vi "Err_Handling.vi"() -> ()   [LabVIEW 2012, in "TB1kW_ErrorProg.lvlib"]
uses:
  TB1kW_ErrorProg.lvlib
  Control and Global/Global_Variables.vi
  Control and Global/Format_Error.ctl
  <vilib>/Utility/error.llb/DialogType.ctl
  <vilib>/Utility/miscctls.llb/LVPointTypeDef.ctl
panel:
  out "Air 100W":bool
  out "O2 100W":bool
  out "H2 CO 100W":bool
  out "N2 100W":bool
  out "H2 100W":bool
  out "MeasErr Array 100W":T1[](array[typedef])
  out "New MesErr file to load 1kW":bool
  out "Last Error/Warning":string
  in  "Show Internal Errors":bool
  out "Watch Dog":bool
  in  "Clear Hist":bool
  out "USV: No 230V":bool
  out "Air":bool
  out "O2":bool
  out "N2":bool
  out "H2":bool
  out "H2 CO":bool
  out "H2 Detected":bool
  out "Em Stop Relay":bool
  out "Em Stop":bool
  out "Error Warning History":string[][](table)
  in  "More/Less":bool
  out "MeasErr Array":T1[](array[typedef])
  in  "Em Stop":bool
  # "Pressure out of range"
  # "Dieser Cluster wird verwendet um das Measurement Error File richtig zu formatieren.\nName: Name des Eingangs, Grösse oder Wertes\nOptions: \n 00: Status des Werts: ok (0), Warnung (-1), Fehler (1)\n 01: Maximaler Wert\n 02: Maximale Dauer in der dieser Wert überschritten werden darf. [s]\n 03: spezifische optionen\nLast Chek at: Zeitpunkt an dem der Wert das letzte Mal geprüft wurde ohne dass ein Limit überschritten wured . Der Zeitpunkt wird nicht mer aktualisiert, falls ein Fehler auftritt so kann die Dauer ermittelt werden."
  # "Dieser Cluster wird verwendet um das Measurement Error File richtig zu formatieren.\nName: Name des Eingangs, Grösse oder Wertes\nOptions: \n 00: Status des Werts: ok (0), Warnung (-1), Fehler (1)\n 01: Maximaler Wert\n 02: Maximale Dauer in der dieser Wert überschritten werden darf. [s]\n 03: spezifische optionen\nLast Chek at: Zeitpunkt an dem der Wert das letzte Mal geprüft wurde ohne dass ein Limit überschritten wured . Der Zeitpunkt wird nicht mer aktualisiert, falls ein Fehler auftritt so kann die Dauer ermittelt werden."
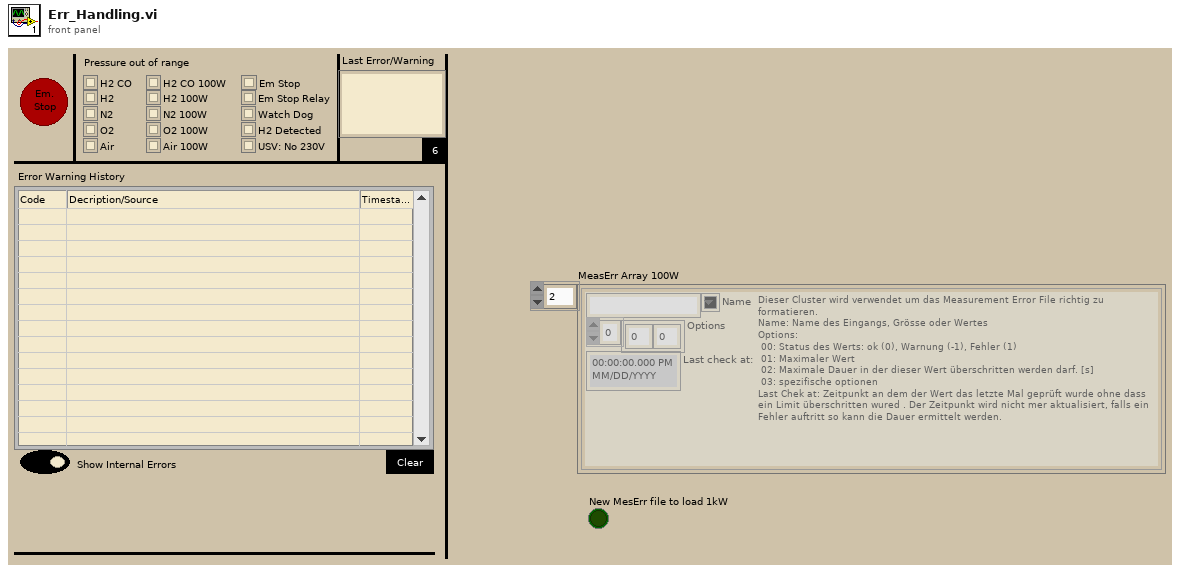
[diagram p1: front panel]
types:
  T1 = typedef "TB1kW_Controls.lvlib/Format_Error.ctl" = cluster{"Name":string, "Options":dbl[], "Last check at:":timestamp}
  T2 = typedef "LVPointTypeDef.ctl" = cluster{"Horizontal":i16, "Vertical":i16}
  T3 = cluster{"Em. Button pressed":bool, "Em. Relay In":bool, "H2 detected":bool, "Watch Dog In":bool, "P_H2 not OK (1)":bool, "P_H2 not OK (2)":bool, "P_N2 not OK (1)":bool, "P_N2 not OK (2)":bool, "P_H2CO not OK (1)":bool, "P_H2CO not OK (2)":bool, "P_O2 not OK (1)":bool, "P_O2 not OK (2)":bool, "P_Air not OK (1)":bool, "P_Air not OK (2)":bool, "I/O 14 MUX":bool, "I/O 15 MUX":bool, "I/O 5":bool, "EM Stop Relay Out":bool, "Watch Dog Out":bool, "USV: No ~230V":bool}
  T4 = cluster{"f1":bool, "f2":bool, "f2":bool, "f3":bool, "New MesErr file to load":bool, "New Command file to load":bool, "f6":bool, "f7":bool, "New MesErr file to load 100W":bool, "New Command file to load 100W":bool}
  T5 = cluster{"Internal Error 1kW":bool, "Test Error 1kW":bool, "Shut down test":bool, "Terminate programm":bool, "Set secure state":bool, "Test is running":bool, "Flush after Error 1kW":bool, "f07":bool, "f08":bool, "Command file created":bool, "f10":bool, "f11":bool, "f12":bool, "f13":bool, "Logging":bool, "Is Measuring Cell Imp.":bool, "Test is running 100W":bool, "Command file created 100W":bool, "Shut down test 100W":bool, "Logging 100W":bool, "Internal Error 100W":bool, "Test Error 100W":bool, "Internal Error":bool, "Set secure state 100W":bool, "Flush after Error 100W":bool, "Init_Dnet":bool, "Use Stopsequenz 1kW":bool, "Use Stopsequenz 100W":bool, "Do Stopsequenz 1kW":bool, "Do Stopsequenz 100W":bool}
  T6 = typedef "Semaphore RefNum" = refnum<k1>
  T7 = typedef "DialogType.ctl" = u16
  T8 = typedef "TB1kW_Controls.lvlib/Test_Properties.ctl" = cluster{"Cell Properties":T9, "Time":T10, "Flow N2 to Ox [Nl/min]":dbl, "Flow N2 to Fuel [Nl/min]":dbl, "Flush time after test error [s]":dbl, "Used Gases":cluster{"H2":bool, "N2":bool, "Air":bool, "O2":bool, "CO H2":bool}, "Fuelcell Temp. [°C]":dbl, "CO mixing ratio in tank [ppm]":dbl, "Stoichiometry Fuel [-]":dbl, "N2 in Fuel [%]":dbl, "Stoichiometry Ox [-]":dbl, "CO in Fuel [ppm]":dbl, "Humidity Ox [%]":dbl, "Humidity Fuel [%]":dbl, "Making I/U Curve":bool, "Meas Cell Impedance":bool, "Imped. Meas Intervall [s]":u32, "Nr. of Comand-Files Rep.":u32, "Use PS1":bool, "Use PS2":bool, "Use cyrostat":bool, "Used Temp Sens":cluster{"Temp 0":bool, "Temp 1":bool, "Temp 2":bool, "Temp 3":bool, "Temp 4":bool, "Temp 5":bool, "Temp 6":bool, "Temp 7":bool}, "Adjust AIn":cluster{"Gain":dbl, "Zero":dbl, "Unit":string}[]}
  T9 = typedef "TB1kW_Controls.lvlib/Cell_Properties.ctl" = cluster{"Nr of cells [-]":u8, "Cell area [cm2]":dbl, "Min. stack voltage [V]":dbl, "Min. cell voltage [mV]":dbl, "Max. stack current [A]":dbl, "Max. Dcell voltage [mV]":dbl, "Last Cell on Pin":i8, "First Cell on Pin":i8}
  T10 = typedef "TB1kW_Controls.lvlib/Time.ctl" = cluster{"[hh:mm:ss]\n[DD/MM/YY]":timestamp, "Include date":bool, "Time used as":string, "[hh:mm:ss]":dbl}
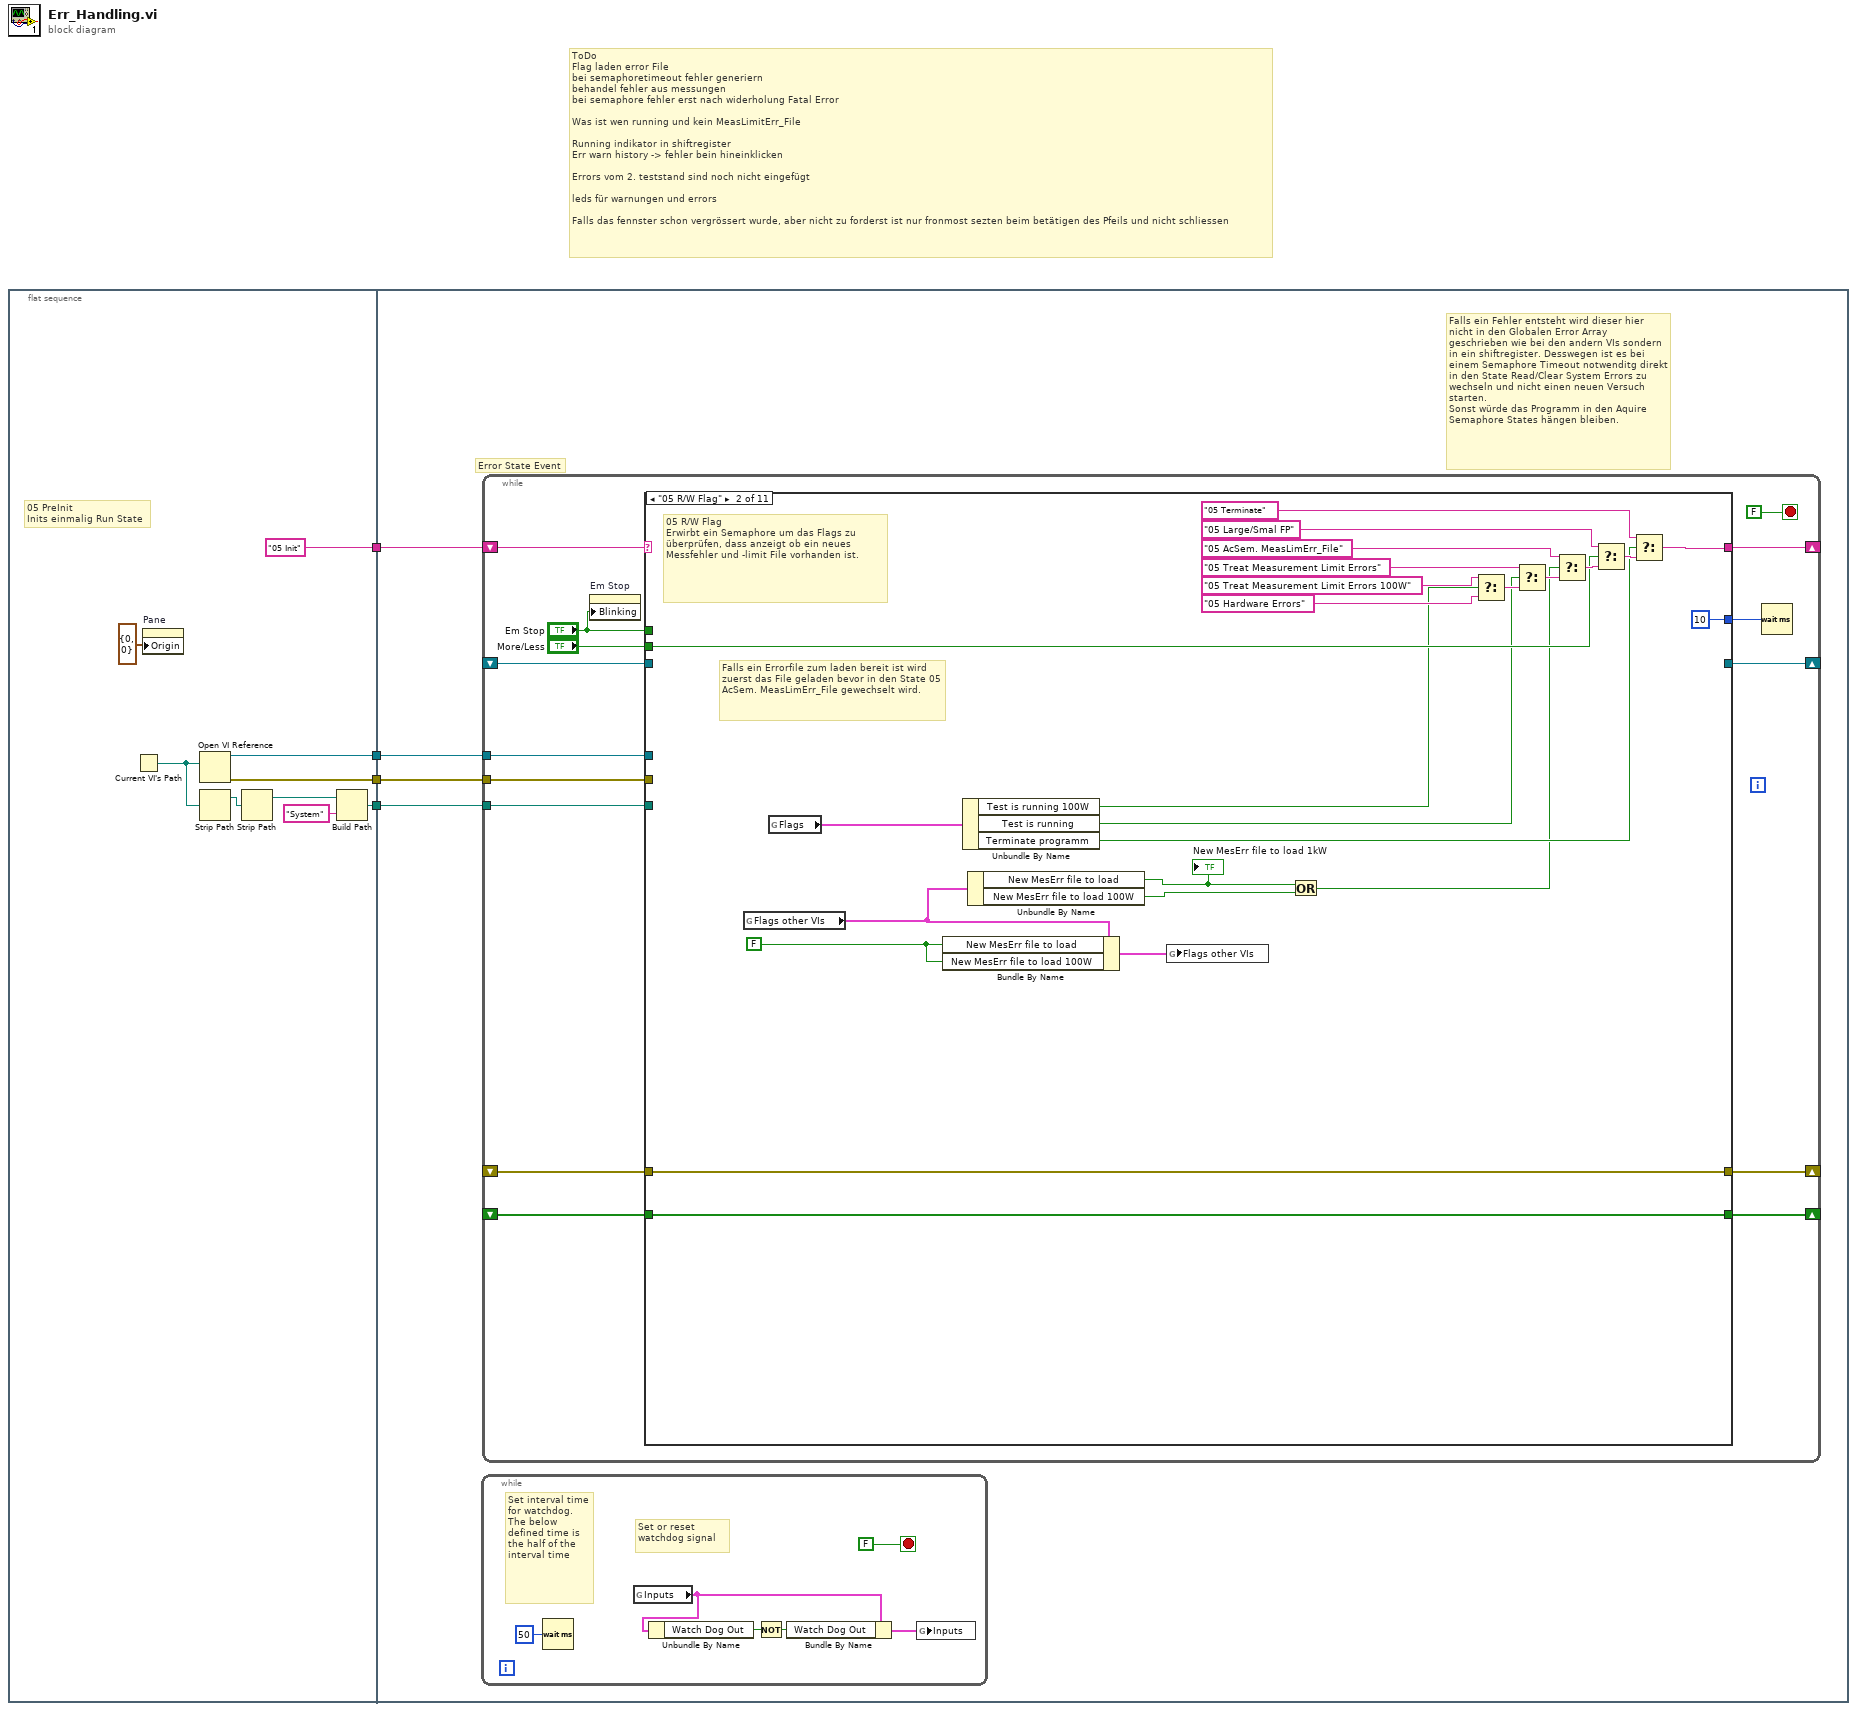
[diagram p0: block diagram]
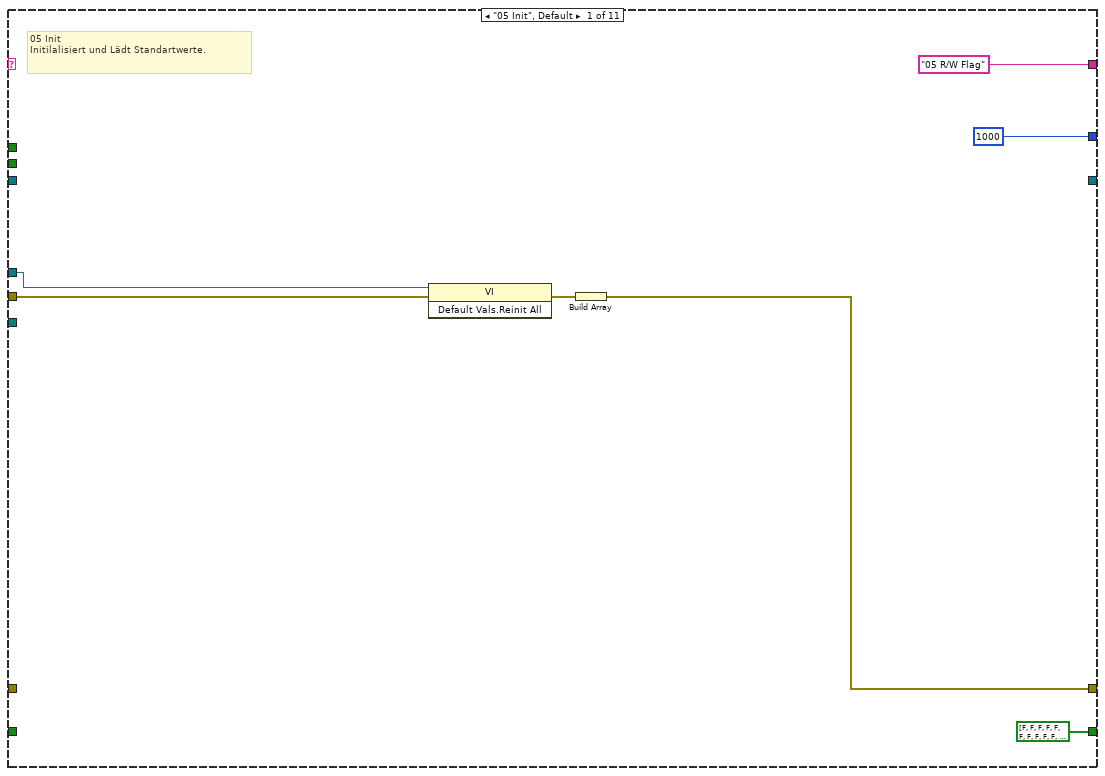
[diagram p2: hidden frame]
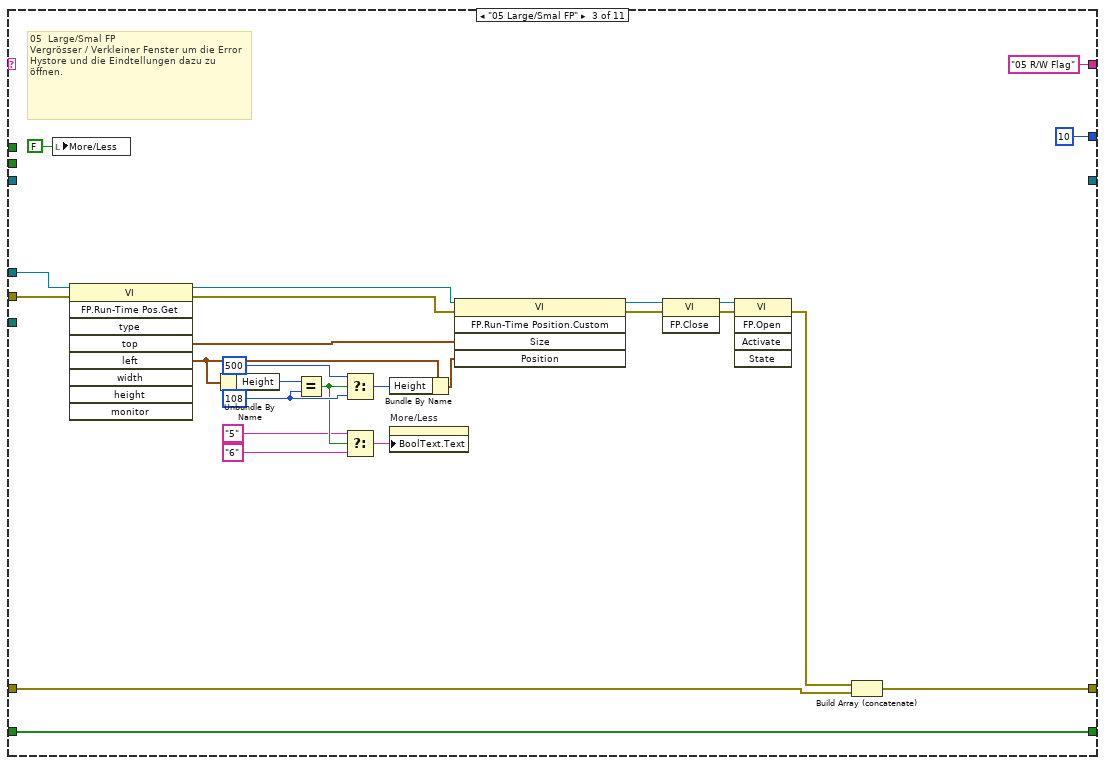
[diagram p3: hidden frame]
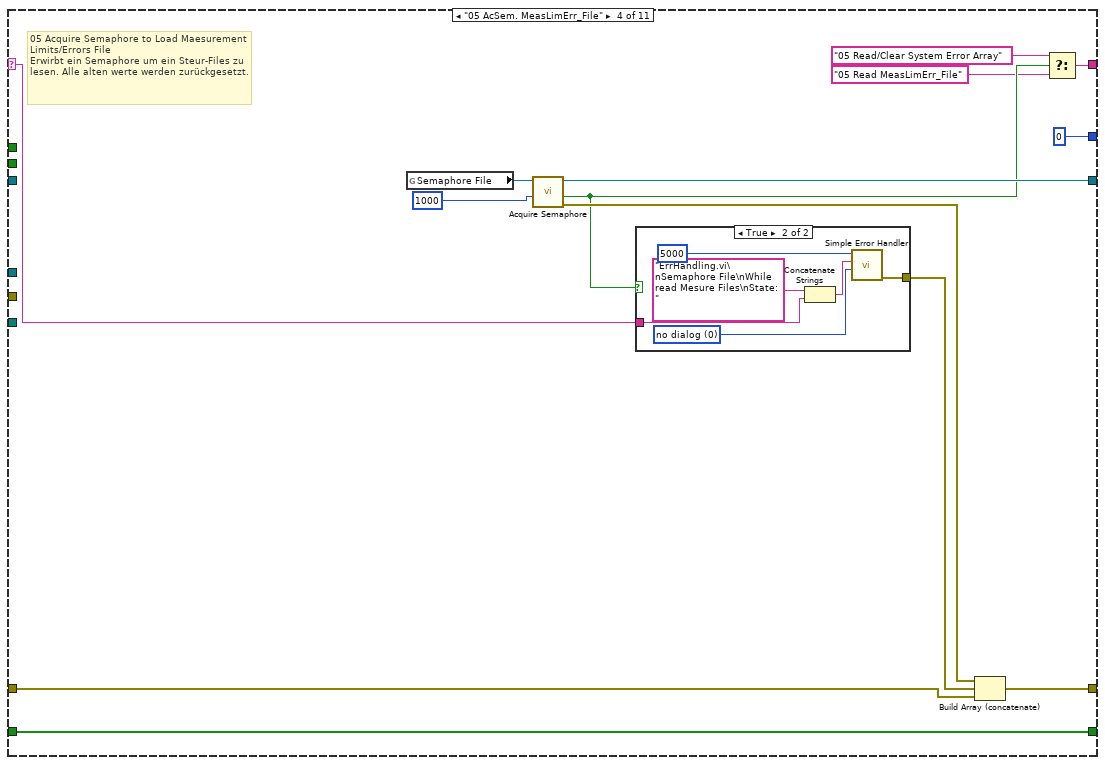
[diagram p4: hidden frame]
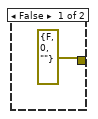
[diagram p5: hidden frame]
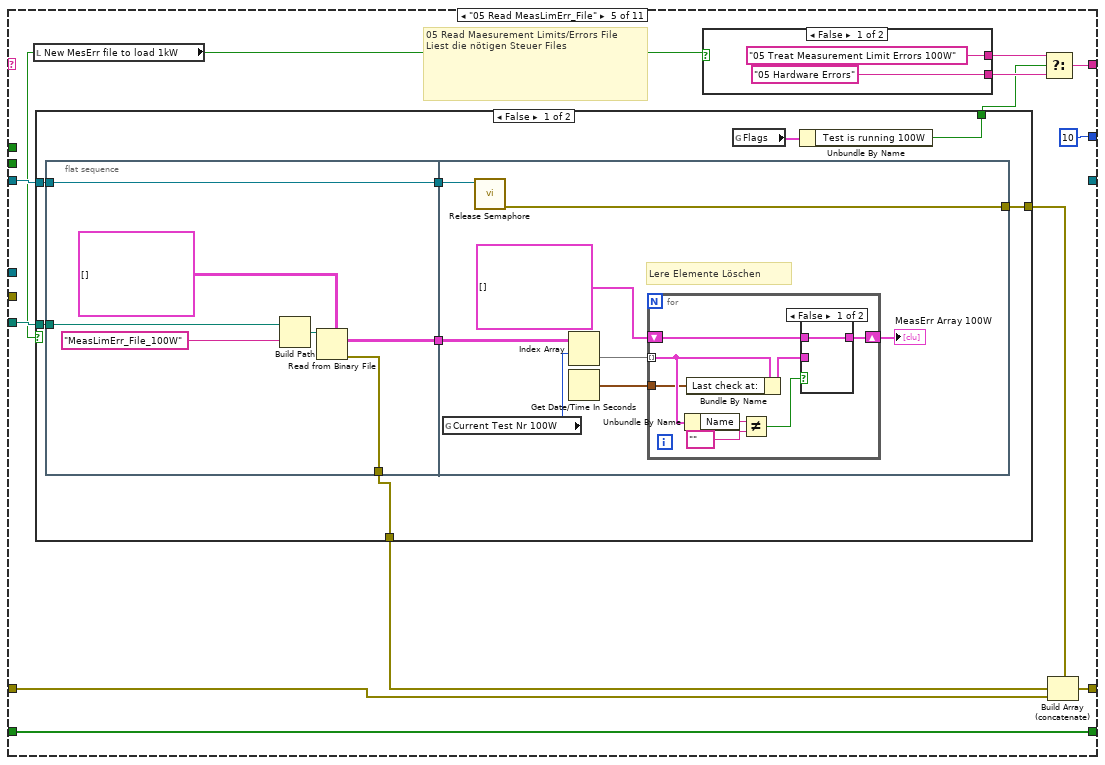
[diagram p6: hidden frame]
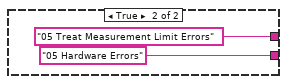
[diagram p7: hidden frame]
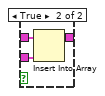
[diagram p8: hidden frame]
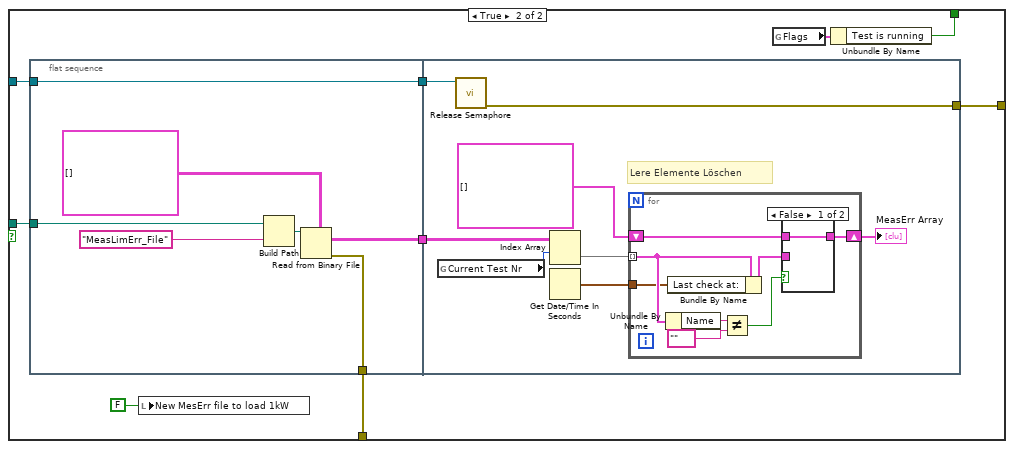
[diagram p9: hidden frame]
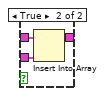
[diagram p10: hidden frame]
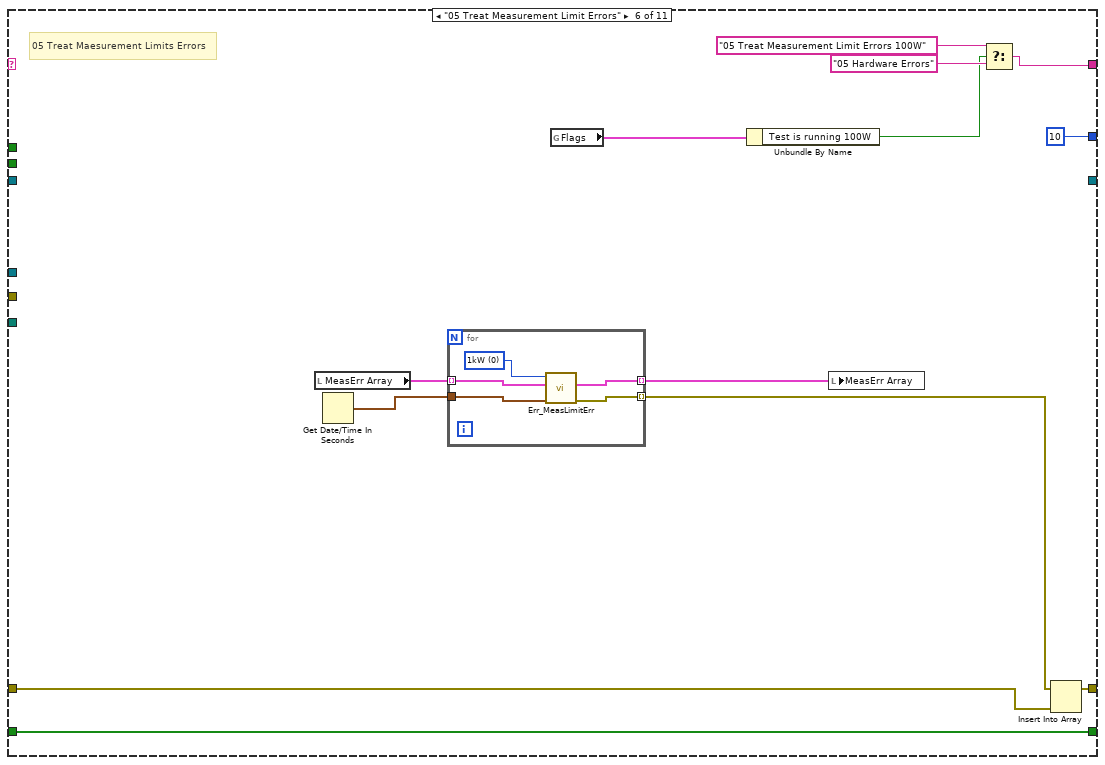
[diagram p11: hidden frame]
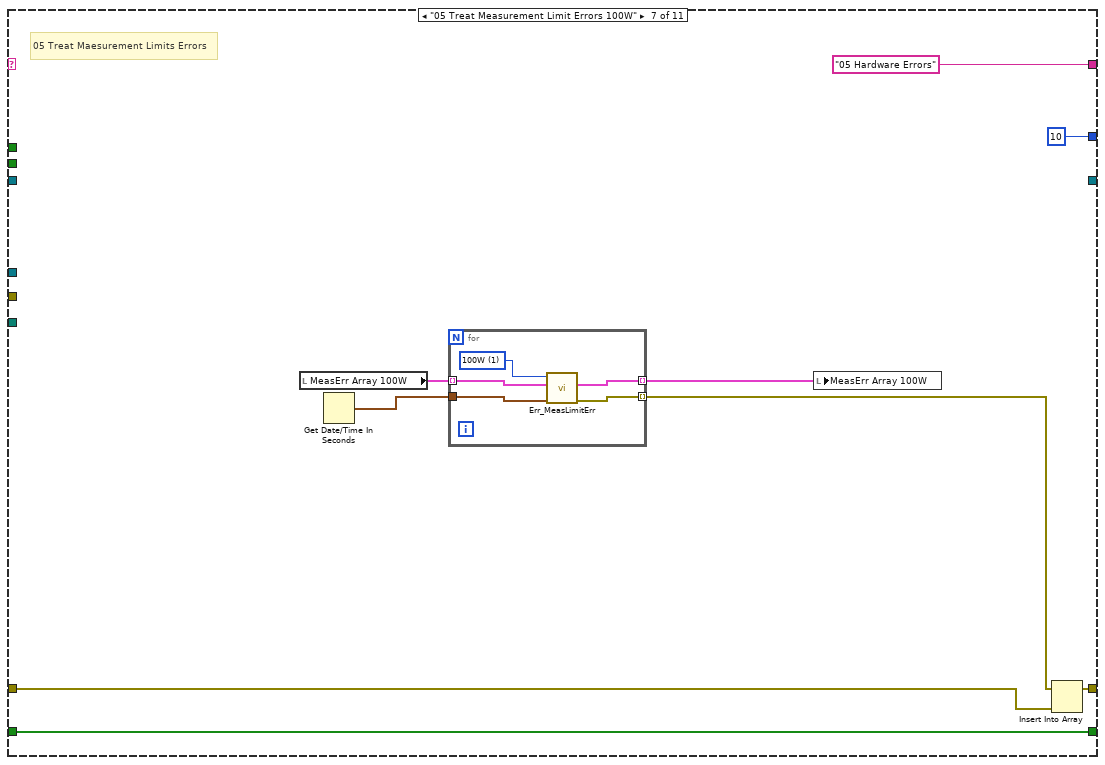
[diagram p12: hidden frame]
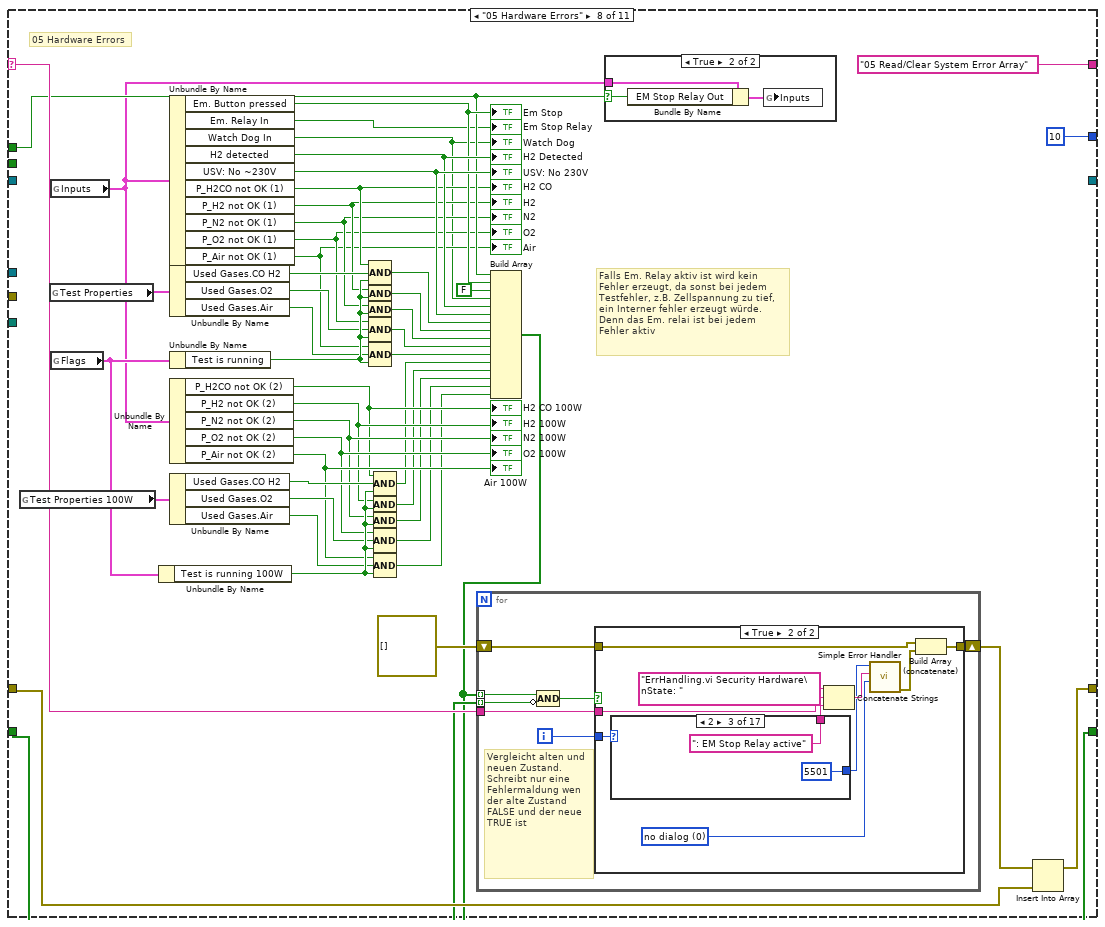
[diagram p13: hidden frame]
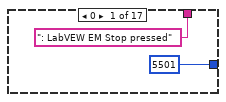
[diagram p16: hidden frame]
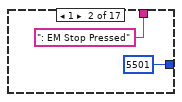
[diagram p17: hidden frame]
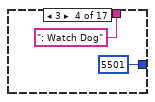
[diagram p18: hidden frame]
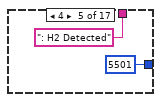
[diagram p19: hidden frame]
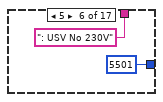
[diagram p20: hidden frame]
diagram:
  # "ToDo\nFlag laden error File\nbei semaphoretimeout fehler generiern\nbehandel fehler aus messungen\nbei semaphore fehler erst nach widerholung Fatal Error\n\nWas ist wen running und kein MeasLimitErr_File\n\nRunning indikator in shiftregister\nErr warn history -> fehler bein hineinklicken\n\nErrors vom 2. teststand sind noch nicht eingefügt\n\nleds für warnungen und errors\n\nFalls das fennster schon vergrössert wurde, aber nicht zu forderst ist nur fronmost sezten beim betätigen des Pfeils und nicht schliessen"
  n1 = flat-sequence {
    tunnel: [w7] -> w4
    tunnel: [w13] -> w3
    tunnel: [w12] -> w2
    tunnel: ["05 Init" ("name or relative path")] -> w1
    tunnel: w4 -> [w15]
    tunnel: w3 -> [w17]
    tunnel: w2 -> [w16]
    tunnel: w1 -> [w14]
    frame #0 {
      # "05 PreInit\nInits einmalig Run State"
      n2 = Current VI's Path() -> (path=w10:path)
      n3 = property on="Pane" class="Pane"("Origin"=T2 {"Horizontal"=0, "Vertical"=0}) -> ()  [unwired: 2 in, 2 out]
      n4 = Open VI Reference(vi path=w10) -> (vi reference=w13:refnum<vi>, error out=w12:errorcluster)  [unwired: 2 in, 3 out]
      n5 = Strip Path(path=w10) -> (stripped path=w11:path)  [unwired: 1 out]
      n6 = Strip Path(path=w11) -> (stripped path=w8:path)  [unwired: 1 out]
      n7 = Build Path(base path=w8, name or relative path="System") -> (appended path=w7:path)
    }
    frame #1 {
      # "Falls ein Fehler entsteht wird dieser hier nicht in den Globalen Error Array geschrieben wie bei den andern VIs sondern in ein shiftregister. Desswegen ist es bei einem Semaphore Timeout notwenditg direkt in den State Read/Clear System Errors zu wechseln und nicht einen neuen Versuch starten.\nSonst würde das Programm in den Aquire Semaphore States hängen bleiben."
      # "Error State Event"
      n8 = while {
        stop <- FALSE stop-if-true
        # "Set interval time for watchdog. The below defined time is the half of the interval time"
        # "Set or reset watchdog signal"
        n9 = Wait (ms)(milliseconds to wait=u32 50 ("Zu wartende ms")) -> ()  [unwired: 1 out]
        n10 = global read "Global_Variables.vi" "Inputs"() -> (w19:T3)
        n11 = Unbundle By Name(w19) -> ("Watch Dog Out"=w21:bool)
        n12 = Not(x=w21) -> (.not. x?=w22:bool)
        n13 = Bundle By Name(cluster=w19, "Watch Dog Out"=w22) -> (w20:T3)
        n14 = global write "Global_Variables.vi" "Inputs"(w20) -> ()
      }
      n15 = while {
        shift-right: [w30] -> _
        shift-left: w14 -> [w28]
        tunnel: w15 -> [w32]
        shift-right: [w36] -> _
        shift-left: _ -> [w35]
        tunnel: w17 -> [w34]
        tunnel: w16 -> [w33]
        shift-right: [w37] -> _
        shift-left: _ -> [w31]
        shift-right: [w26] -> _
        shift-left: _ -> [w25]
        stop <- FALSE stop-if-true
        n16 = property on="Em Stop" class="Bool (strict)"("Blinking"="Em Stop") -> ()  [unwired: 2 in, 2 out]
        n17 = case shown="\"05 R/W Flag\"" w28 {
          selector: w28 -> [_ _ _ w104 _ _ _ w283 _ _ _]
          tunnel: ["05 R/W Flag" w57 "05 R/W Flag" w110 w123 w206 "05 Hardware Errors" "05 Read/Clear System Error Array" "05 Treat All Errors" "05 R/W Flag" "05 Terminate"] -> w30
          tunnel: [u32 1000 ("milliseconds to wait") u32 10 ("milliseconds to wait") u32 10 ("milliseconds to wait") u32 0 ("milliseconds to wait") u32 10 ("milliseconds to wait") u32 10 ("milliseconds to wait") u32 10 ("milliseconds to wait") u32 10 ("milliseconds to wait") u32 10 ("milliseconds to wait") u32 10 ("milliseconds to wait") u32 10 ("milliseconds to wait")] -> w29
          tunnel: w32 -> [_ _ _ _ w128 _ _ _ _ _ _]
          tunnel: w35 -> [_ _ _ _ w129 _ _ _ _ _ _]
          tunnel: w34 -> [w42 _ w87 _ _ _ _ _ _ _ w433]
          tunnel: w33 -> [w43 _ w86 _ _ _ _ _ _ _ w432]
          tunnel: [_ _ _ w103 _ _ _ _ _ _ _] -> w36
          tunnel: [w41 w68 w89 w100 w127 w213 w227 w256 w343 errorcluster[] [] w429] -> w37
          tunnel: w31 -> [_ w68 w90 w101 w125 w214 w226 w258 w344 w355 w428]
          tunnel: "More/Less" -> [_ w61 _ _ _ _ _ _ _ _ _]
          tunnel: "Em Stop" -> [_ _ _ _ _ _ _ w270 _ _ _]
          tunnel: [bool[] [FALSE, FALSE, FALSE, FALSE, FALSE, FALSE, FALSE, FALSE, FALSE, FALSE, FALSE, FALSE, FALSE, FALSE, FALSE, FALSE, FALSE, FALSE, FALSE, FALSE, FALSE] w59 w71 w97 w120 w211 w228 w238 w341 w352 w426] -> w26
          tunnel: w25 -> [_ w59 w71 w97 w120 w211 w228 w257 w341 w352 w426]
          frame "05 Init", Default {
            # "05 Init\nInitilalisiert und Lädt Standartwerte."
            n18 = invoke class="VI" method="Default Vals.Reinit All"(reference=w42, error in=w43) -> (error out=w44:errorcluster)  [unwired: 1 in, 2 out]
            n19 = Build Array(w44) -> (w41:errorcluster[])
          }
          frame "05 R/W Flag" {
            w51 = FALSE ("Measurement error file created")
            # "Falls ein Errorfile zum laden bereit ist wird zuerst das File geladen bevor in den State 05 AcSem. MeasLimErr_File gewechselt wird."
            # "05 R/W Flag\nErwirbt ein Semaphore um das Flags zu überprüfen, dass anzeigt ob ein neues Messfehler und -limit File vorhanden ist."
            n20 = global read "Global_Variables.vi" "Flags other VIs"() -> (w66:T4)
            n21 = global read "Global_Variables.vi" "Flags"() -> (w67:T5)
            n22 = Bundle By Name(cluster=w66, "New MesErr file to load"=w51, "New MesErr file to load 100W"=w51) -> (w65:T4)
            n23 = Unbundle By Name(w67) -> ("Test is running 100W"=w47:bool, "Test is running"=w46:bool, "Terminate programm"=w55:bool)
            n24 = Unbundle By Name(w66) -> ("New MesErr file to load"=w54:bool, "New MesErr file to load 100W"=w53:bool)
            "New MesErr file to load 1kW" <- w54
            n25 = global write "Global_Variables.vi" "Flags other VIs"(w65) -> ()
            n26 = Or(x=w54, y=w53) -> (x .or. y?=w52:bool)
            n27 = Select(t="05 Treat Measurement Limit Errors 100W", s=w47, f="05 Hardware Errors") -> (s? t:f=w50:string)
            n28 = Select(t="05 Treat Measurement Limit Errors", s=w46, f=w50) -> (s? t:f=w69:string)
            n29 = Select(t="05 AcSem. MeasLimErr_File", s=w52, f=w69) -> (s? t:f=w62:string)
            n30 = Select(t="05 Large/Smal FP", s=w61, f=w62) -> (s? t:f=w56:string)
            n31 = Select(t="05 Terminate", s=w55, f=w56) -> (s? t:f=w57:string)
          }
          frame "05 Large/Smal FP" {
            w93 = i16 108 ("y")
            # "05  Large/Smal FP\nVergrösser / Verkleiner Fenster um die Error Hystore und die Eindtellungen dazu zu öffnen."
            n32 = local write "More/Less"(FALSE ("More/Less")) -> ()
            n33 = invoke class="VI" method="FP.Run-Time Pos.Get"(reference=w87, error in=w86) -> (reference out=w84:refnum<vi>, error out=w83:errorcluster, "top"=w81:cluster{"Top":i16, "Left":i16}, "left"=w85:cluster{"Height":i16, "Width":i16})  [unwired: 7 in, 5 out]
            n34 = Unbundle By Name(w85) -> ("Height"=w94:i16)
            n35 = Equal?(x=w94, y=w93) -> (x = y?=w75:bool)
            n36 = Select(t=i16 500 ("y"), s=w75, f=w93) -> (s? t:f=w91:i16)
            n37 = Select(t="5", s=w75, f="6") -> (s? t:f=w72:string)
            n38 = Bundle By Name(cluster=w85, "Height"=w91) -> (w82:cluster{"Height":i16, "Width":i16})
            n39 = property on="More/Less" class="Bool (strict)"("BoolText.Text"=w72) -> ()  [unwired: 2 in, 2 out]
            n40 = invoke class="VI" method="FP.Run-Time Position.Custom"(reference=w84, error in=w83, "Size"=w81, "Position"=w82) -> (reference out=w79:refnum<vi>, error out=w78:errorcluster)  [unwired: 1 in, 3 out]
            n41 = invoke class="VI" method="FP.Close"(reference=w79, error in=w78) -> (reference out=w76:refnum<vi>, error out=w77:errorcluster)  [unwired: 1 in, 1 out]
            n42 = invoke class="VI" method="FP.Open"(reference=w76, error in=w77) -> (error out=w80:errorcluster)  [unwired: 3 in, 4 out]
            n43 = Build Array (concatenate)(w80, w90) -> (w89:errorcluster[])
          }
          frame "05 AcSem. MeasLimErr_File" {
            # "05 Acquire Semaphore to Load Maesurement Limits/Errors File\nErwirbt ein Semaphore um ein Steur-Files zu lesen. Alle alten werte werden zurückgesetzt."
            n44 = global read "Global_Variables.vi" "Semaphore File"() -> (w107:T6)
            n45 = call <vilib>:"Acquire Semaphore.vi"("ms timeout (-1)"=1000, "semaphore"=w107) -> ("error out"=w106:errorcluster, "timed out"=w102:bool, "semaphore out"=w103:T6)  [unwired: 1 in, 2 out]
            n46 = case shown="True" w102 {
              tunnel: [errorcluster {"status"=FALSE, "code"=0, "source"=""} ("error out") w115] -> w105
              tunnel: w104 -> [_ w112]
              frame False {
              }
              frame True {
                w116 = T7 0 items=["no dialog", "OK message", "continue or stop message", "OK message + warnings", "continue/stop + warnings"] ("type of dialog (OK msg:1)")
                n47 = Concatenate Strings("ErrHandling.vi\nSemaphore File\nWhile read Mesure Files\nState: " ("error source (\" \")"), w112) -> (w113:string)
                n48 = call <vilib>:"Simple Error Handler.vi"("error code (no error:0)"=5000, "error source (\" \")"=w113, "type of dialog (OK msg:1)"=w116) -> ("error out"=w115:errorcluster)  [unwired: 1 in, 5 out]
              }
            }
            n49 = Build Array (concatenate)(w106, w105, w101) -> (w100:errorcluster[])
            n50 = Select(t="05 Read/Clear System Error Array", s=w102, f="05 Read MeasLimErr_File") -> (s? t:f=w110:string)
          }
          frame "05 Read MeasLimErr_File" {
            # "05 Read Maesurement Limits/Errors File\nLiest die nötigen Steuer Files"
            n51 = local read "New MesErr file to load 1kW"() -> (w119:bool)
            n52 = case shown="False" w119 {
              tunnel: w129 -> [w140 w176]
              tunnel: w128 -> [w139 w175]
              tunnel: [w136 w174] -> w126
              tunnel: [w135 w173] -> w124
              tunnel: [w137 w170] -> w118
              frame False {
                n53 = flat-sequence {
                  tunnel: [w144] -> w142
                  tunnel: [w148] -> w141
                  tunnel: [w146] -> w135
                  tunnel: w140 -> [w144]
                  tunnel: w139 -> [w143]
                  tunnel: w142 -> [w157]
                  tunnel: w141 -> [w156]
                  tunnel: [w155] -> w136
                  frame #0 {
                    n54 = Build Path(base path=w143, name or relative path="MeasLimErr_File_100W") -> (appended path=w149:path)
                    n55 = Read from Binary File(5:T1[][] [] ("appended array"), 11:w149) -> (0:w146:errorcluster, 2:w148:T1[][])  [unwired: 1 in, 5 out]
                  }
                  frame #1 {
                    # "Lere Elemente Löschen"
                    n56 = global read "Global_Variables.vi" "Current Test Nr 100W"() -> (w153:i32)
                    n57 = call <vilib>:"Release Semaphore.vi"("semaphore"=w157) -> ("error out"=w155:errorcluster)  [unwired: 1 in, 5 out]
                    n58 = Index Array(array=w156, index (row)=w153) -> (element=w154:T1[])  [unwired: 1 in]
                    n59 = Get Date/Time In Seconds() -> (seconds since 1Jan1904=w150:timestamp)
                    n60 = for {
                      tunnel: w154 -> [w160] mode=indexing
                      shift-right: [w163] -> w152
                      shift-left: T1[] [] -> [w162]
                      tunnel: w150 -> [w158]
                      n61 = Unbundle By Name(w160) -> ("Name"=w165:string)
                      n62 = Bundle By Name(cluster=w160, "Last check at:"=w158) -> (w159:T1)
                      n63 = Not Equal?(x=w165, y="" ("Name")) -> (x != y?=w161:bool)
                      n64 = case shown="False" w161 {
                        tunnel: [w166 w169] -> w163
                        tunnel: w159 -> [_ w168]
                        tunnel: w162 -> [w166 w167]
                        frame False {
                        }
                        frame True {
                          n65 = Insert Into Array(array=w167, new element=w168) -> (w169:T1[])  [unwired: 1 in]
                        }
                      }
                    }
                    "MeasErr Array 100W" <- w152
                  }
                }
                n66 = global read "Global_Variables.vi" "Flags"() -> (w138:T5)
                n67 = Unbundle By Name(w138) -> ("Test is running 100W"=w137:bool)
              }
              frame True {
                n68 = flat-sequence {
                  tunnel: w176 -> [w185]
                  tunnel: [w185] -> w178
                  tunnel: w175 -> [w182]
                  tunnel: [w183] -> w177
                  tunnel: [w180] -> w173
                  tunnel: w178 -> [w193]
                  tunnel: w177 -> [w192]
                  tunnel: [w191] -> w174
                  frame #0 {
                    n69 = Build Path(base path=w182, name or relative path="MeasLimErr_File") -> (appended path=w184:path)
                    n70 = Read from Binary File(5:T1[][] [] ("appended array"), 11:w184) -> (0:w180:errorcluster, 2:w183:T1[][])  [unwired: 1 in, 5 out]
                  }
                  frame #1 {
                    # "Lere Elemente Löschen"
                    n71 = global read "Global_Variables.vi" "Current Test Nr"() -> (w189:i32)
                    n72 = call <vilib>:"Release Semaphore.vi"("semaphore"=w193) -> ("error out"=w191:errorcluster)  [unwired: 1 in, 5 out]
                    n73 = Index Array(array=w192, index (row)=w189) -> (element=w190:T1[])  [unwired: 1 in]
                    n74 = Get Date/Time In Seconds() -> (seconds since 1Jan1904=w186:timestamp)
                    n75 = for {
                      tunnel: w190 -> [w196] mode=indexing
                      shift-right: [w199] -> w188
                      shift-left: T1[] [] -> [w198]
                      tunnel: w186 -> [w194]
                      n76 = Unbundle By Name(w196) -> ("Name"=w201:string)
                      n77 = Bundle By Name(cluster=w196, "Last check at:"=w194) -> (w195:T1)
                      n78 = Not Equal?(x=w201, y="" ("Name")) -> (x != y?=w197:bool)
                      n79 = case shown="False" w197 {
                        tunnel: [w202 w205] -> w199
                        tunnel: w195 -> [_ w204]
                        tunnel: w198 -> [w202 w203]
                        frame False {
                        }
                        frame True {
                          n80 = Insert Into Array(array=w203, new element=w204) -> (w205:T1[])  [unwired: 1 in]
                        }
                      }
                    }
                    "MeasErr Array" <- w188
                  }
                }
                n81 = local write "New MesErr file to load 1kW"(FALSE ("New MesErr file to load 1kW")) -> ()
                n82 = global read "Global_Variables.vi" "Flags"() -> (w171:T5)
                n83 = Unbundle By Name(w171) -> ("Test is running"=w170:bool)
              }
            }
            n84 = case shown="False" w119 {
              tunnel: ["05 Treat Measurement Limit Errors 100W" "05 Treat Measurement Limit Errors"] -> w122
              tunnel: ["05 Hardware Errors" "05 Hardware Errors"] -> w121
              frame False {
              }
              frame True {
              }
            }
            n85 = Select(t=w122, s=w118, f=w121) -> (s? t:f=w123:string)
            n86 = Build Array (concatenate)(w126, w124, w125) -> (w127:errorcluster[])
          }
          frame "05 Treat Measurement Limit Errors" {
            # "05 Treat Maesurement Limits Errors"
            n87 = local read "MeasErr Array"() -> (w217:T1[])
            n88 = Get Date/Time In Seconds() -> (seconds since 1Jan1904=w212:timestamp)
            n89 = for {
              tunnel: w217 -> [w221] mode=indexing
              tunnel: [w223] -> w216 mode=indexing
              tunnel: [w222] -> w215 mode=indexing
              tunnel: w212 -> [w220]
              w219 = u8 0 items=["1kW", "100W"] ("Testbench")
              n90 = call "Err_MeasLimitErr.vi"("Current time"=w220, "Measurement Error Limit In"=w221, "Testbench"=w219) -> ("Error out"=w222:errorcluster, "Measurement Error Limit Out"=w223:T1)  [unwired: 3 out]
            }
            n91 = global read "Global_Variables.vi" "Flags"() -> (w210:T5)
            n92 = Unbundle By Name(w210) -> ("Test is running 100W"=w207:bool)
            n93 = local write "MeasErr Array"(w216) -> ()
            n94 = Select(t="05 Treat Measurement Limit Errors 100W", s=w207, f="05 Hardware Errors") -> (s? t:f=w206:string)
            n95 = Insert Into Array(array=w215, new element=w214) -> (w213:errorcluster[])  [unwired: 1 in]
          }
          frame "05 Treat Measurement Limit Errors 100W" {
            # "05 Treat Maesurement Limits Errors"
            n96 = local read "MeasErr Array 100W"() -> (w232:T1[])
            n97 = Get Date/Time In Seconds() -> (seconds since 1Jan1904=w229:timestamp)
            n98 = for {
              tunnel: w232 -> [w235] mode=indexing
              tunnel: [w237] -> w231 mode=indexing
              tunnel: [w236] -> w230 mode=indexing
              tunnel: w229 -> [w234]
              w233 = u8 1 items=["1kW", "100W"] ("Testbench")
              n99 = call "Err_MeasLimitErr.vi"("Current time"=w234, "Measurement Error Limit In"=w235, "Testbench"=w233) -> ("Error out"=w236:errorcluster, "Measurement Error Limit Out"=w237:T1)  [unwired: 3 out]
            }
            n100 = local write "MeasErr Array 100W"(w231) -> ()
            n101 = Insert Into Array(array=w230, new element=w226) -> (w227:errorcluster[])  [unwired: 1 in]
          }
          frame "05 Hardware Errors" {
            # "Falls Em. Relay aktiv ist wird kein Fehler erzeugt, da sonst bei jedem Testfehler, z.B. Zellspannung zu tief, ein Interner fehler erzeugt würde. Denn das Em. relai ist bei jedem Fehler aktiv"
            # "05 Hardware Errors"
            n102 = global read "Global_Variables.vi" "Test Properties 100W"() -> (w255:T8)
            n103 = global read "Global_Variables.vi" "Test Properties"() -> (w278:T8)
            n104 = global read "Global_Variables.vi" "Inputs"() -> (w239:T3)
            n105 = global read "Global_Variables.vi" "Flags"() -> (w250:T5)
            n106 = Unbundle By Name(w250) -> ("Test is running 100W"=w253:bool)
            n107 = Unbundle By Name(w239) -> ("Em. Button pressed"=w271:bool, "Em. Relay In"=→"Em Stop Relay":bool, "Watch Dog In"=w264:bool, "H2 detected"=w272:bool, "USV: No ~230V"=w273:bool, "P_H2CO not OK (1)"=w269:bool, "P_H2 not OK (1)"=w268:bool, "P_N2 not OK (1)"=w267:bool, "P_O2 not OK (1)"=w266:bool, "P_Air not OK (1)"=w265:bool)
            "H2 Detected" <- w272
            "H2" <- w268
            "N2" <- w267
            "Em Stop" <- w271
            "H2 CO" <- w269
            "O2" <- w266
            "Air" <- w265
            "USV: No 230V" <- w273
            "Watch Dog" <- w264
            n108 = Unbundle By Name(w278) -> ("Used Gases.CO H2"=w277:bool, "Used Gases.O2"=w275:bool, "Used Gases.Air"=w274:bool)
            n109 = Unbundle By Name(w250) -> ("Test is running"=w276:bool)
            n110 = Unbundle By Name(w239) -> ("P_H2CO not OK (2)"=w245:bool, "P_H2 not OK (2)"=w246:bool, "P_N2 not OK (2)"=w247:bool, "P_O2 not OK (2)"=w248:bool, "P_Air not OK (2)"=w249:bool)
            "H2 100W" <- w246
            "N2 100W" <- w247
            "H2 CO 100W" <- w245
            "O2 100W" <- w248
            "Air 100W" <- w249
            n111 = Unbundle By Name(w255) -> ("Used Gases.CO H2"=w254:bool, "Used Gases.O2"=w252:bool, "Used Gases.Air"=w251:bool)
            n112 = And(x=w268, y=w276) -> (x .and. y?=w259:bool)
            n113 = And(x=w267, y=w276) -> (x .and. y?=w261:bool)
            n114 = Compound Arithmetic op=AND(w269, w277, w276) -> (w260:bool)
            n115 = Compound Arithmetic op=AND(w266, w275, w276) -> (w280:bool)
            n116 = Compound Arithmetic op=AND(w265, w274, w276) -> (w279:bool)
            n117 = And(x=w246, y=w253) -> (x .and. y?=w243:bool)
            n118 = And(x=w247, y=w253) -> (x .and. y?=w242:bool)
            n119 = Compound Arithmetic op=AND(w245, w254, w253) -> (w244:bool)
            n120 = Compound Arithmetic op=AND(w248, w252, w253) -> (w241:bool)
            n121 = Compound Arithmetic op=AND(w249, w251, w253) -> (w240:bool)
            n122 = Build Array(w270, w271, FALSE ("Element"), w264, w272, w273, w260, w259, w261, w280, w279, w244, w243, w242, w241, w240) -> (w238:bool[])
            n123 = for {
              tunnel: w238 -> [w294] mode=indexing
              tunnel: w257 -> [w295] mode=indexing
              shift-right: [w293] -> w281
              shift-left: errorcluster[] [] -> [w292]
              tunnel: w283 -> [w289]
              i -> [w290]
              # "Vergleicht alten und neuen Zustand.\nSchreibt nur eine Fehlermaldung wen der alte Zustand FALSE und der neue TRUE ist"
              n124 = Compound Arithmetic op=AND(w294, invert w295) -> (w291:bool)
              n125 = case shown="True" w291 {
                tunnel: [w296 w300] -> w293
                tunnel: w292 -> [w296 w302]
                tunnel: w290 -> [_ w299]
                tunnel: w289 -> [_ w303]
                frame False {
                }
                frame True {
                  w306 = T7 0 items=["no dialog", "OK message", "continue or stop message", "OK message + warnings", "continue/stop + warnings"] ("type of dialog (OK msg:1)")
                  n126 = case shown="2" w299 {
                    tunnel: [": LabVEW EM Stop pressed" ("error source (\" \")") ": EM Stop Pressed" ("error source (\" \")") ": EM Stop Relay active" ("error source (\" \")") ": Watch Dog" ("error source (\" \")") ": H2 Detected" ("error source (\" \")") ": USV No 230V" ("error source (\" \")") ": Pressure H2 CO out of range" ("error source (\" \")") ": Pressure H2 out of range" ("error source (\" \")") ": Pressure N2 out of range" ("error source (\" \")") ": Pressure O2 out of range" ("error source (\" \")") ": Pressure Air out of range" ("error source (\" \")") ": Pressure H2 CO 100W out of range" ("error source (\" \")") ": Pressure H2 100W out of range" ("error source (\" \")") ": Pressure N2 100W out of range" ("error source (\" \")") ": Pressure O2 100W out of range" ("error source (\" \")") ": Pressure Air 100W out of range" ("error source (\" \")") ": Input not known " ("error source (\" \")")] -> w298
                    tunnel: [5501 ("error code (no error:0)") 5501 ("error code (no error:0)") 5501 ("error code (no error:0)") 5501 ("error code (no error:0)") 5501 ("error code (no error:0)") 5501 ("error code (no error:0)") 5502 ("error code (no error:0)") 5502 ("error code (no error:0)") 5502 ("error code (no error:0)") 5502 ("error code (no error:0)") 5502 ("error code (no error:0)") 5503 ("error code (no error:0)") 5503 ("error code (no error:0)") 5503 ("error code (no error:0)") 5503 ("error code (no error:0)") 5503 ("error code (no error:0)") 5501 ("error code (no error:0)")] -> w297
                    frame 0 {
                    }
                    frame 1 {
                    }
                    frame 2 {
                    }
                    frame 3 {
                    }
                    frame 4 {
                    }
                    frame 5 {
                    }
                    frame 6 {
                    }
                    frame 7 {
                    }
                    frame 8 {
                    }
                    frame 9 {
                    }
                    frame 10 {
                    }
                    frame 11 {
                    }
                    frame 12 {
                    }
                    frame 13 {
                    }
                    frame 14 {
                    }
                    frame 15 {
                    }
                    frame 21, Default {
                    }
                  }
                  n127 = Concatenate Strings("ErrHandling.vi Security Hardware\nState: " ("error source (\" \")"), w303, w298) -> (w304:string)
                  n128 = call <vilib>:"Simple Error Handler.vi"("error code (no error:0)"=w297, "error source (\" \")"=w304, "type of dialog (OK msg:1)"=w306) -> ("error out"=w301:errorcluster)  [unwired: 1 in, 5 out]
                  n129 = Build Array (concatenate)(w302, w301) -> (w300:errorcluster[])
                }
              }
            }
            n130 = case shown="True" w270 {
              selector: w270 -> [_ w286]
              tunnel: w239 -> [_ w287]
              frame False {
              }
              frame True {
                n131 = Bundle By Name(cluster=w287, "EM Stop Relay Out"=w286) -> (w288:T3)
                n132 = global write "Global_Variables.vi" "Inputs"(w288) -> ()
              }
            }
            n133 = Insert Into Array(array=w281, new element=w258) -> (w256:errorcluster[])  [unwired: 1 in]
          }
          frame "05 Read/Clear System Error Array" {
            # "05 Read and Clear System Error Array\nLiest den System Error Array aus und fügt ihn mit den anderen Fehlern zusammen um diese danach zu beareuiten. Der System Error Array wird danach gelöscht"
            n134 = flat-sequence {
              tunnel: [w347] -> w345
              frame #0 {
                n135 = global read "Global_Variables.vi" "Errors"() -> (w347:errorcluster[])
              }
              frame #1 {
                n136 = global write "Global_Variables.vi" "Errors"(errorcluster[] []) -> ()
              }
            }
            n137 = Insert Into Array(array=w345, new element=w344) -> (w343:errorcluster[])  [unwired: 1 in]
          }
          frame "05 Treat All Errors" {
            # "05 Treat All Errors\nHier werden alle Fehler behandelt\nund die im gesamten System auftretn"
            n138 = case shown="True" "Clear Hist" {
              tunnel: [w359 string[][] []] -> w350
              frame False {
                n139 = local read "Error Warning History"() -> (w359:string[][])
              }
              frame True {
                n140 = local write "Last Error/Warning"("" ("Last Error/Warning")) -> ()
              }
            }
            n141 = Get Date/Time In Seconds() -> (seconds since 1Jan1904=w354:timestamp)
            n142 = for {
              tunnel: w355 -> [w367] mode=indexing
              tunnel: w354 -> [w366]
              shift-right: [w362] -> w353
              shift-left: w350 -> [w363]
              tunnel: "Show Internal Errors" -> [w365]
              n143 = Unbundle By Name(w367) -> ("code"=w368:i32)
              n144 = case shown="5501" w368 {
                tunnel: w367 -> [_ _ _ _ _ _ _ _ w408 w415 w420]
                tunnel: [_ TRUE ("Fatal Error") _ w396 w399 _ _ _ TRUE ("Fatal Error") TRUE ("Fatal Error") TRUE ("Fatal Error")] -> w364
                frame 0, Default {
                }
                frame -8501, -8500 {
                }
                frame 5000 {
                  # "Semaphore Time out"
                }
                frame 6000..6006 {
                  w396 = TRUE ("Fatal Error")
                  # "Test Errors"
                  n145 = global read "Global_Variables.vi" "Flags"() -> (w397:T5)
                  n146 = Bundle By Name(cluster=w397, "Test Error 1kW"=w396) -> (w398:T5)
                  n147 = global write "Global_Variables.vi" "Flags"(w398) -> ()
                }
                frame 6007..6013 {
                  w399 = TRUE ("Fatal Error")
                  # "Test Errors"
                  n148 = global read "Global_Variables.vi" "Flags"() -> (w401:T5)
                  n149 = Bundle By Name(cluster=w401, "Test Error 100W"=w399) -> (w400:T5)
                  n150 = global write "Global_Variables.vi" "Flags"(w400) -> ()
                }
                frame 5011 {
                  # "Unable to write Error"
                  n151 = global read "Global_Variables.vi" "Flags"() -> (w402:T5)
                  n152 = Bundle By Name(cluster=w402, "Internal Error 100W"=TRUE ("Fatal Error")) -> (w403:T5)
                  n153 = global write "Global_Variables.vi" "Flags"(w403) -> ()
                }
                frame 5010 {
                  # "Unable to write output"
                  n154 = global read "Global_Variables.vi" "Flags"() -> (w407:T5)
                  n155 = Bundle By Name(cluster=w407, "Internal Error 1kW"=TRUE ("Fatal Error")) -> (w406:T5)
                  n156 = global write "Global_Variables.vi" "Flags"(w406) -> ()
                }
                frame 5012 {
                }
                frame 5501 {
                  # "Security hardware error"
                  n157 = Unbundle By Name(w408) -> ()  [unwired: 2 out]
                  n158 = case shown="True" TRUE {
                    frame False {
                    }
                    frame True {
                      n159 = global read "Global_Variables.vi" "Flags"() -> (w413:T5)
                      n160 = Bundle By Name(cluster=w413, "Internal Error"=TRUE ("Fatal Error")) -> (w412:T5)
                      n161 = global write "Global_Variables.vi" "Flags"(w412) -> ()
                    }
                  }
                }
                frame 5502 {
                  # "Security hardware error"
                  n162 = Unbundle By Name(w415) -> ()  [unwired: 2 out]
                  n163 = case shown="True" TRUE {
                    frame False {
                    }
                    frame True {
                      n164 = global read "Global_Variables.vi" "Flags"() -> (w419:T5)
                      n165 = Bundle By Name(cluster=w419, "Internal Error 1kW"=TRUE ("Fatal Error")) -> (w418:T5)
                      n166 = global write "Global_Variables.vi" "Flags"(w418) -> ()
                    }
                  }
                }
                frame 5503 {
                  # "Security hardware error"
                  n167 = Unbundle By Name(w420) -> ()  [unwired: 2 out]
                  n168 = case shown="True" TRUE {
                    frame False {
                    }
                    frame True {
                      n169 = global read "Global_Variables.vi" "Flags"() -> (w425:T5)
                      n170 = Bundle By Name(cluster=w425, "Internal Error 100W"=TRUE ("Fatal Error")) -> (w424:T5)
                      n171 = global write "Global_Variables.vi" "Flags"(w424) -> ()
                    }
                  }
                }
              }
              n172 = case shown="Error" w367 {
                selector: w367 -> [_ w378]
                tunnel: w363 -> [w369 w375]
                tunnel: [w369 w374] -> w362
                tunnel: w366 -> [_ w377]
                tunnel: w365 -> [_ w372]
                tunnel: w364 -> [_ w371]
                frame No Error {
                }
                frame Error {
                  n173 = Unbundle By Name(w378) -> ("code"=w376:i32, "source"=w373:string)
                  n174 = Or(x=w371, y=w372) -> (x .or. y?=w370:bool)
                  n175 = case shown="True" w370 {
                    tunnel: w377 -> [_ w394]
                    tunnel: w376 -> [_ w392]
                    tunnel: w375 -> [w379 w391]
                    tunnel: [w379 w390] -> w374
                    tunnel: w373 -> [_ w382]
                    frame False {
                    }
                    frame True {
                      w384 = ": " ("String")
                      n176 = Get Date/Time String(date format (0)=enum16{"short", "long", "abbreviated"}."long", seconds (now)=w394, want seconds? (F)=TRUE) -> (date string=w387:string, time string=w386:string)
                      n177 = Number To Decimal String(number=w392) -> (decimal integer string=w385:string)  [unwired: 1 out]
                      n178 = Concatenate Strings(w386, "\r", w387) -> (w383:string)
                      n179 = Build Array(w385, w382, w383) -> (w380:string[])
                      n180 = Concatenate Strings(w385, w384, w382, w384, w383, w384) -> (→"Last Error/Warning":string)
                      n181 = Build Array (concatenate)(w380, w391) -> (w390:string[][])
                    }
                  }
                }
              }
            }
            "Error Warning History" <- w353
          }
          frame "05 Terminate" {
            # "(Wird nicht mehr ausgeführt)"
            # "05 Terminate"
            n182 = invoke class="VI" method="FP.Close"(reference=w433, error in=w432) -> (reference out=w430:refnum<vi>, error out=w431:errorcluster)  [unwired: 1 in, 1 out]
            n183 = invoke class="VI" method="Abort VI"(reference=w430, error in=w431) -> (error out=w434:errorcluster)  [unwired: 1 in, 2 out]
            n184 = Build Array (concatenate)(w434, w428) -> (w429:errorcluster[])
          }
        }
        n185 = Wait (ms)(milliseconds to wait=w29) -> ()  [unwired: 1 out]
      }
    }
  }
